vi "Configure OSC Limit Open.vi"(8 "error in (no error)":errorcluster, 9 "Limit Open":dbl=0.1 min=0.1 max=1.0 step=0.1 format="%.1f", 10 "Step":T1=1 min=1 max=99 step=1, 11 "VISA resource name":refnum<visa-resource-name>) -> (0 "error out":errorcluster, 3 "VISA resource name out":refnum<visa-resource-name>)   [LabVIEW 2025, in "Chroma 19052.lvlib"]
uses:
  <instrlib>/Chroma 19052/Public/Utility/Type Def/steps--numeric.ctl
  <instrlib>/Chroma 19052/Chroma 19052.lvlib
panel:
  # "Configure OSC Limit Open"
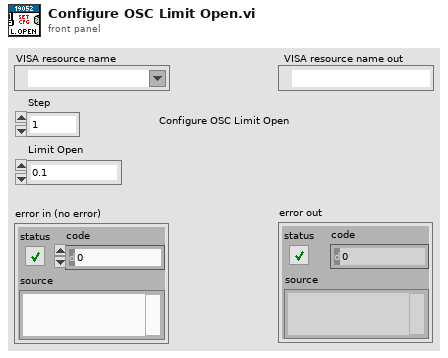
[diagram p1: front panel]
types:
  T1 = typedef "Chroma 19052.lvlib/steps--numeric.ctl" = u8
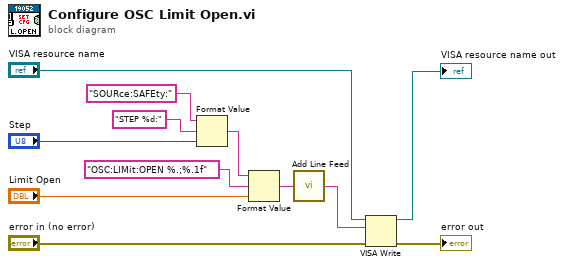
[diagram p0: block diagram]
diagram:
  n1 = Format Value(string ("")="SOURce:SAFEty:", format string="STEP %d:", value (0)="Step") -> (output string=w1:string)
  n2 = Format Value(string ("")=w1, format string="OSC:LIMit:OPEN %.;%.1f", value (0)="Limit Open") -> (output string=w7:string)
  n3 = call <instrlib>:"Add Line Feed.vi"("Command string"=w7) -> ("Concatenated string"=w6:string)  [unwired: 4 in]
  n4 = VISA Write(VISA resource name="VISA resource name", write buffer=w6, error in (no error)="error in (no error)") -> (VISA resource name out=→"VISA resource name out":refnum<visa-resource-name>, error out=→"error out":errorcluster)  [unwired: 1 out]
